vi "FlipFlop.vi"() -> ()   [LabVIEW 2020]
panel:
  out "Array":dbl[][](array[numeric])
  in  "stop":bool
  out "Waveform Graph":dbl[][](graph)
  out "rand":dbl
  out "let output":bool
  in  "min":dbl
  in  "max":dbl
  # "se  generan los numeros aleatorios y pasan por el control de maximos y minimos, cuando quiera deterner la generacion de numeros presione stop\ny en ese momento se presentará la grafica y la tabla de valores para constatar el funcionamiento."
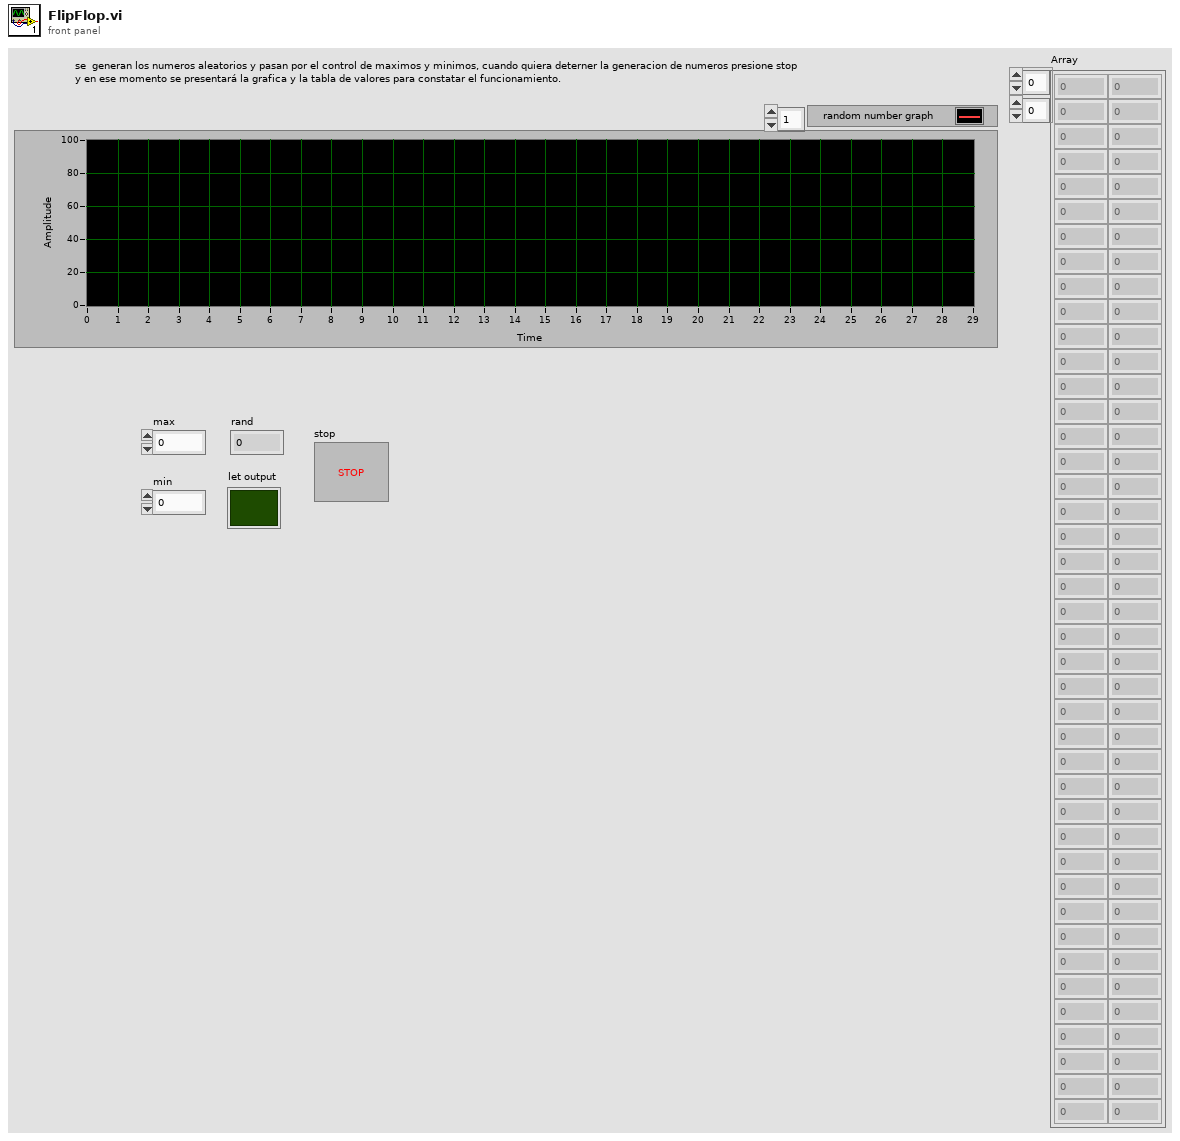
[diagram p1: front panel]
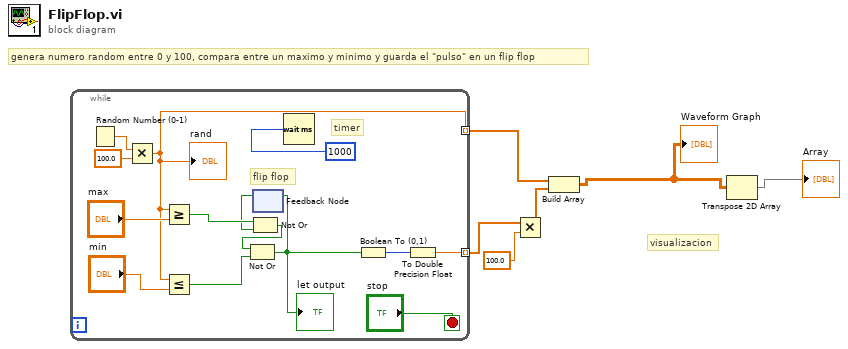
[diagram p0: block diagram]
diagram:
  # "visualizacion"
  # "genera numero random entre 0 y 100, compara entre un maximo y minimo y guarda el \"pulso\" en un flip flop"
  n1 = while {
    tunnel: [w9] -> w4 mode=indexing
    tunnel: [w8] -> w6 mode=indexing
    stop <- "stop" stop-if-true
    # "timer"
    # "flip flop"
    n2 = Random Number (0-1)() -> (number: 0 to 1=w20:dbl)
    n3 = Multiply(x=w20, y=100.0) -> (x*y=w8:dbl)
    "rand" <- w8
    n4 = Greater Or Equal?(x=w8, y="max") -> (x >= y?=w16:bool)
    n5 = Less Or Equal?(x=w8, y="min") -> (x <= y?=w17:bool)
    n6 = feedback #1() -> (w13:bool)  [unwired: 1 in]
    n7 = Not Or(1:w13, 2:w16) -> (0:w12:bool)
    n8 = Not Or(1:w17, 2:w12) -> (0:w11:bool)
    "let output" <- w11
    n9 = feedback-in #1(w11) -> ()
    n10 = Wait (ms)(milliseconds to wait=u32 1000) -> ()  [unwired: 1 out]
    n11 = Boolean To (0,1)(Boolean=w11) -> (0, 1=w10:i16)
    n12 = To Double Precision Float(number=w10) -> (double precision float=w9:dbl)
  }
  n13 = Multiply(x=w4, y=100.0) -> (x*y=w3:dbl[])
  n14 = Build Array(w6, w3) -> (w2:dbl[][])
  "Waveform Graph" <- w2
  n15 = Transpose 2D Array(2D array=w2) -> (transposed array=→"Array":dbl[][])
